vi "Close.vi"(8 "error in (no error)":errorcluster, 11 "TIFF Writer in":refnum<class "TIFF Writer.lvclass">) -> (0 "error out":errorcluster, 3 "path":path)   [LabVIEW 2020, in "LV Tiff.lvlib" / "TIFF Writer.lvclass"]
uses:
  TIFF Writer.lvclass
  TIFF Writer.lvclass/TIFF Writer.ctl
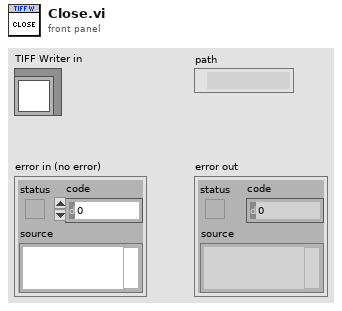
[diagram p1: front panel]
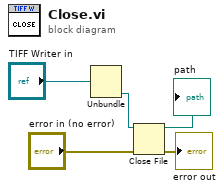
[diagram p0: block diagram]
diagram:
  n1 = Unbundle("TIFF Writer in") -> (w2:refnum<file>)  [unwired: 3 out]
  n2 = Close File(refnum=w2, error in="error in (no error)") -> (path=→"path":path, error out=→"error out":errorcluster)
